vi "Write.vi"(8 "error in":errorcluster, 9 "Producer Ch":T2, 10 "Producer Control":T1, 11 "Chiller Cluster.lvclass":refnum<class "Chiller Cluster.lvclass">) -> (0 "error out":errorcluster, 3 "output cluster":refnum<class "Chiller Cluster.lvclass">)   [LabVIEW 2023, in "Chiller Cluster.lvclass"]
uses:
  Chiller Cluster.lvclass
  6bfc6677-cd67-4f2d-afef-839dec9218ce.vi
  74f11eb1-9425-41af-a169-6608e4aa6674.vi
  Producer Ch Array.ctl
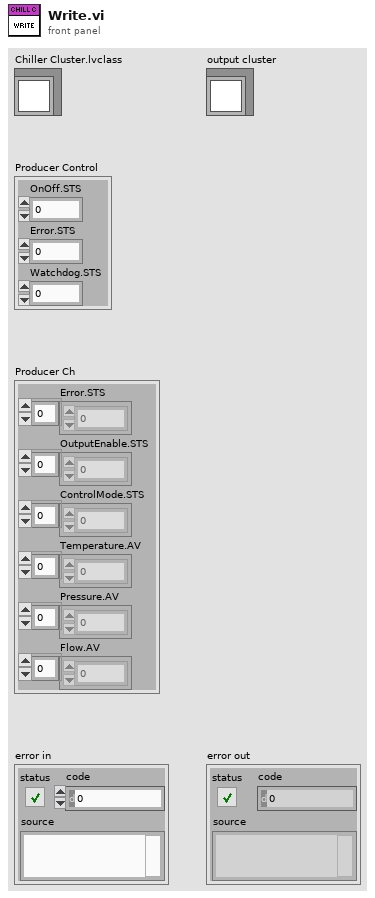
[diagram p1: front panel]
types:
  T1 = cluster{"OnOff.STS":i32, "Error.STS":i32, "Watchdog.STS":i32}
  T2 = typedef "Chiller Cluster.lvclass/Producer Ch Array.ctl" = cluster{"Error.STS":i32[], "OutputEnable.STS":i32[], "ControlMode.STS":u16[], "Temperature.AV":dbl[], "Pressure.AV":dbl[], "Flow.AV":dbl[]}
  T3 = cluster{"Error.STS":i32, "OutputEnable.STS":i32, "ControlMode.STS":u16, "Temperature.AV":dbl, "Pressure.AV":dbl, "Flow.AV":dbl}
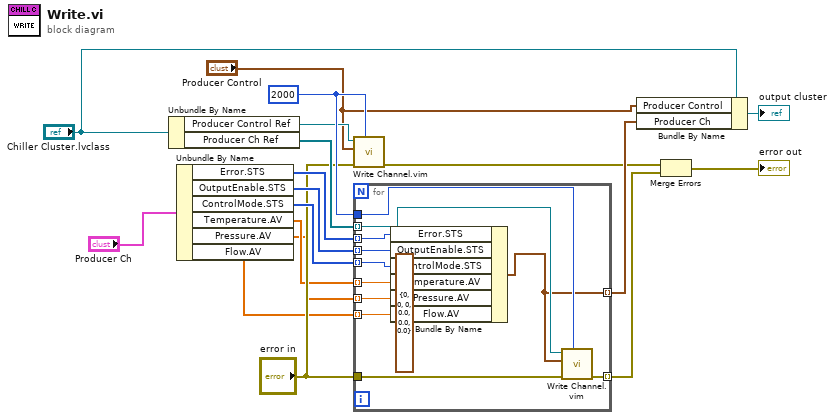
[diagram p0: block diagram]
diagram:
  w11 = 2000 ("Timeout (ms)")
  n1 = Unbundle By Name("Chiller Cluster.lvclass") -> ("Producer Control Ref"=w10:refnum<k21>, "Producer Ch Ref"=w12:refnum<k21>[])
  n2 = Unbundle By Name("Producer Ch") -> ("Error.STS"=w17:i32[], "OutputEnable.STS"=w16:i32[], "ControlMode.STS"=w15:u16[], "Temperature.AV"=w4:dbl[], "Pressure.AV"=w3:dbl[], "Flow.AV"=w2:dbl[])
  n3 = call "Write Channel.vim"("Timeout (ms)"=w11, "error in"="error in", "Data in"="Producer Control", "ADAS HIL Channel in"=w10) -> ("error out"=w7:errorcluster)  [unwired: 5 in, 2 out]
  n4 = for {
    tunnel: w17 -> [w19] mode=indexing
    tunnel: w16 -> [w20] mode=indexing
    tunnel: w15 -> [w21] mode=indexing
    tunnel: [w25] -> w9 mode=indexing
    tunnel: "error in" -> [w30]
    tunnel: [w29] -> w6 mode=indexing
    tunnel: w12 -> [w28] mode=indexing
    tunnel: w11 -> [w27]
    tunnel: w4 -> [w24] mode=indexing
    tunnel: w3 -> [w23] mode=indexing
    tunnel: w2 -> [w22] mode=indexing
    n5 = Bundle By Name(cluster=T3 {"Error.STS"=0, "OutputEnable.STS"=0, "ControlMode.STS"=0, "Temperature.AV"=0.0, "Pressure.AV"=0.0, "Flow.AV"=0.0} ("Producer Ch"), "Error.STS"=w19, "OutputEnable.STS"=w20, "ControlMode.STS"=w21, "Temperature.AV"=w24, "Pressure.AV"=w23, "Flow.AV"=w22) -> (w25:T3)
    n6 = call "Write Channel.vim"("Timeout (ms)"=w27, "error in"=w30, "Data in"=w25, "ADAS HIL Channel in"=w28) -> ("error out"=w29:errorcluster)  [unwired: 5 in, 2 out]
  }
  n7 = Bundle By Name(cluster="Chiller Cluster.lvclass", "Producer Control"="Producer Control", "Producer Ch"=w9) -> (→"output cluster":refnum<class "Chiller Cluster.lvclass">)
  n8 = Merge Errors(w7, w6) -> (→"error out":errorcluster)
